vi "Close All References.vi"(8 "error in (no error)":errorcluster, 11 "Filled Text Fields Actor in":refnum<class "Filled Text Fields Actor.lvclass">) -> (0 "error out":errorcluster, 3 "Filled Text Fields Actor out":refnum<class "Filled Text Fields Actor.lvclass">)   [LabVIEW 2017, in "Filled Text Fields.lvlib" / "Filled Text Fields Actor.lvclass"]
uses:
  Filled Text Fields Actor.lvclass
  Filled Text Fields Actor.lvclass/Filled Text Fields Actor.ctl
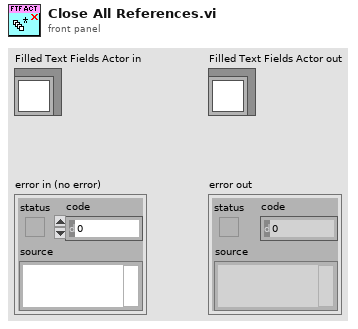
[diagram p1: front panel]
types:
  T1 = typedef "Filled Text Fields.lvlib/Filled Text Fields Actor.lvclass/Filled Text Fields.Events.ctl" = cluster{"stopChanged":refnum<user-event>, "New Value":refnum<user-event>}
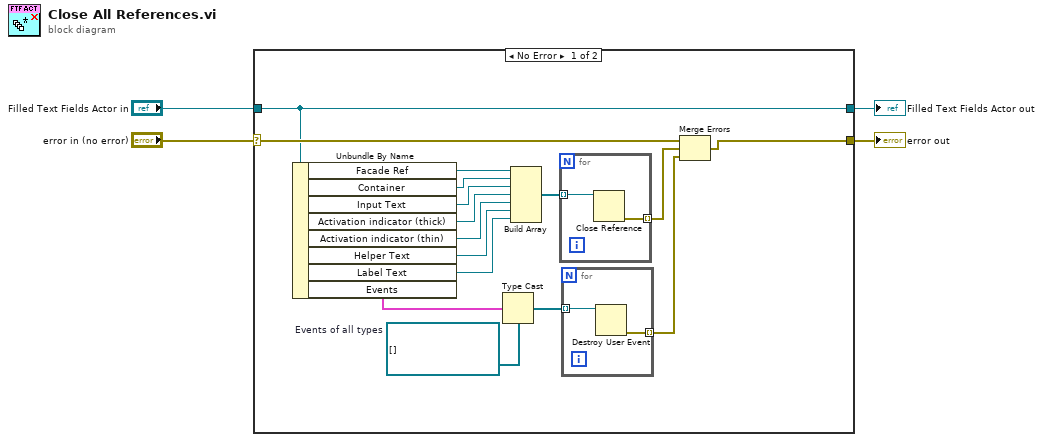
[diagram p0: block diagram]
diagram:
  n1 = case shown="No Error" "error in (no error)" {
    selector: "error in (no error)" -> [w20 w26]
    tunnel: [w10 w26] -> w3
    tunnel: [w19 w25] -> w1
    tunnel: "Filled Text Fields Actor in" -> [w19 w25]
    frame No Error {
      w7 = refnum<user-event>[] []  # Events of all types
      n2 = Unbundle By Name(w19) -> ("Facade Ref"=w18:refnum<vi>, "Container"=w17:refnum<vi>, "Input Text"=w16:refnum<vi>, "Activation indicator (thick)"=w15:refnum<vi>, "Activation indicator (thin)"=w14:refnum<vi>, "Helper Text"=w13:refnum<vi>, "Label Text"=w12:refnum<vi>, "Events"=w8:T1)
      n3 = Type Cast(type=w7, x=w8) -> (*(type *) &x=w6:refnum<user-event>[])
      n4 = Build Array(w18, w17, w16, w15, w14, w13, w12) -> (w11:refnum<vi>[])
      n5 = for {
        tunnel: w11 -> [w24] mode=indexing
        tunnel: [w23] -> w9 mode=indexing
        n6 = Close Reference(reference=w24) -> (error out=w23:errorcluster)  [unwired: 1 in]
      }
      n7 = for {
        tunnel: w6 -> [w22] mode=indexing
        tunnel: [w21] -> w5 mode=indexing
        n8 = Destroy User Event(user event=w22) -> (error out=w21:errorcluster)  [unwired: 1 in]
      }
      n9 = Merge Errors(w20, w9, w5) -> (w10:errorcluster)
    }
    frame Error {
    }
  }
  "error out" <- w3
  "Filled Text Fields Actor out" <- w1
